vi "SDCP - Standard Message Frames Editor - Main.vi"() -> ()   [LabVIEW 2020]
uses:
  Typedefs/SDCP - Standard Message Frames Editor - Parameter cluster.ctl
panel:
  in  "Transmit tick (us)":dbl
  in  "Transmit code file path":path
  in  "Generator transmit code":bool
  in  "Load Excel File":bool
  in  "Source Excel file path":path
  in  "Destination Parameter file path":path
  in  "Parameter list":i32(listbox)
  in  "Parameter index":i32
  in  "Stop application":bool
  in  "Source Parameter file path":path
  in  "C code file path":path
  in  "Load parameter file":bool
  in  "Generate Parameter File":bool
  in  "Generate C code":bool
  in  "Frame ID":i32
  in  "Frame Name":string
  in  "Delete Parameter":bool
  in  "Frame details":T2(array[cluster])
  in  "Delete frame":bool
  in  "Add Frame":bool
  # "Frame Details"
  # "Note: \nValid data types for \nparameters are \nunsigned, signed and\nfloat."
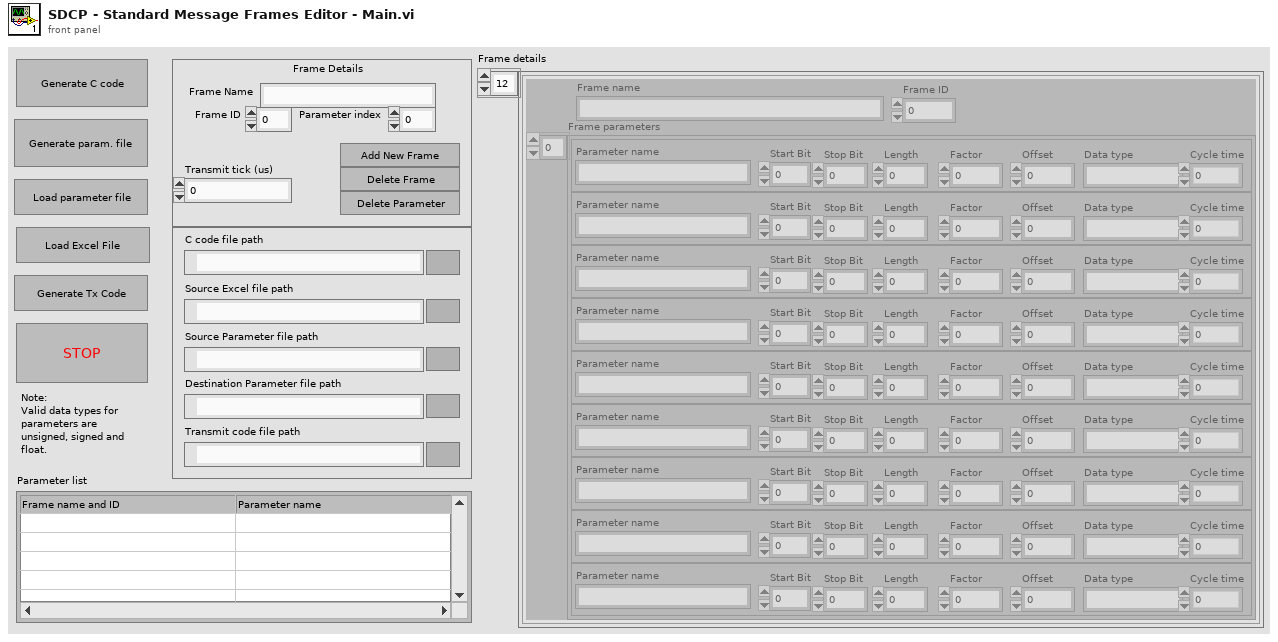
[diagram p1: front panel]
types:
  T1 = typedef "SDCP - Standard Message Frames Editor - Parameter cluster.ctl" = cluster{"Parameter name":string, "Start Bit":i32, "Stop Bit":i32, "Length":i32, "Factor":dbl, "Offset":dbl, "Data type":string, "Cycle time":dbl}
  T2 = cluster{"Frame name":string, "Frame ID":i32, "Frame parameters":T1[]}[]
  T3 = cluster{"Frame name":string, "Frame ID":i32, "Frame parameters":T1[]}
  T4 = enum16{"open", "replace", "create", "open or create", "replace or create", "replace or create with confirmation"}
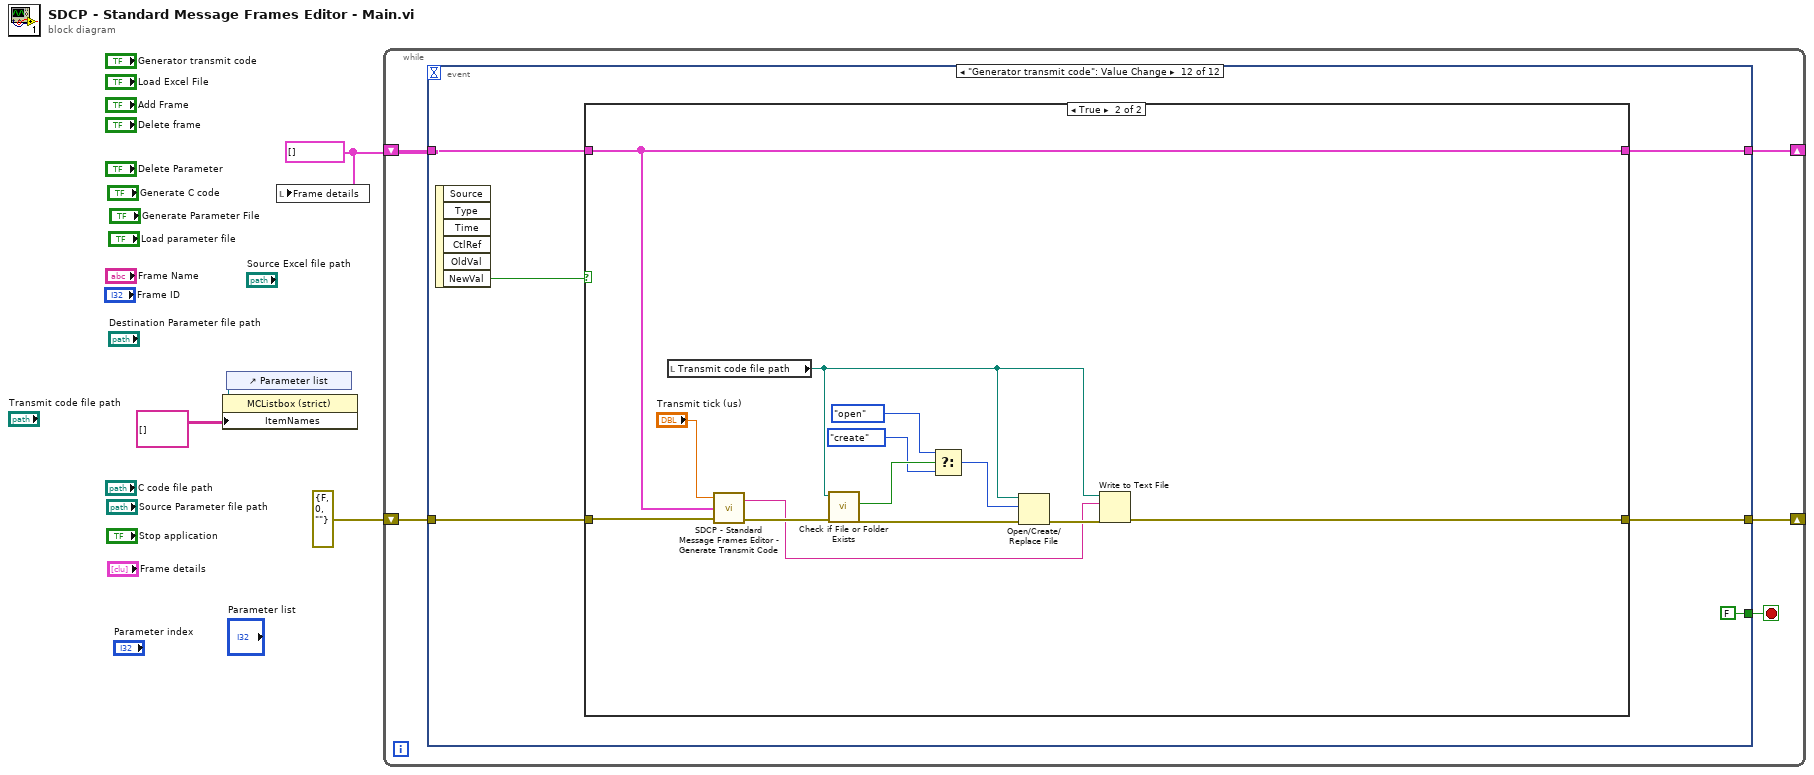
[diagram p0: block diagram]
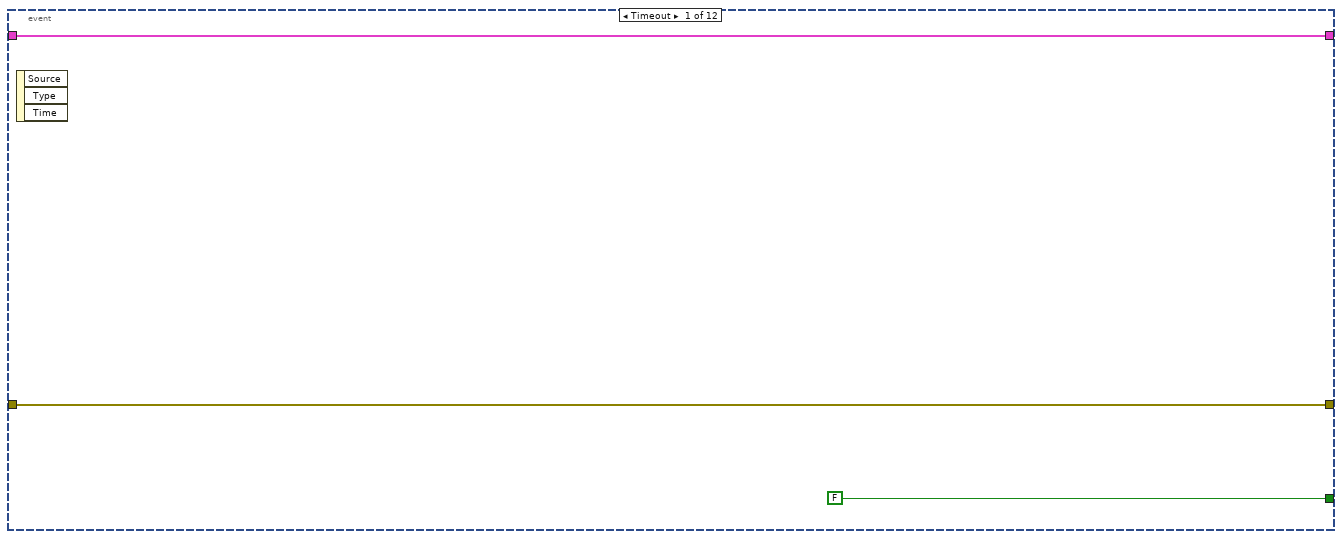
[diagram p2: hidden frame]
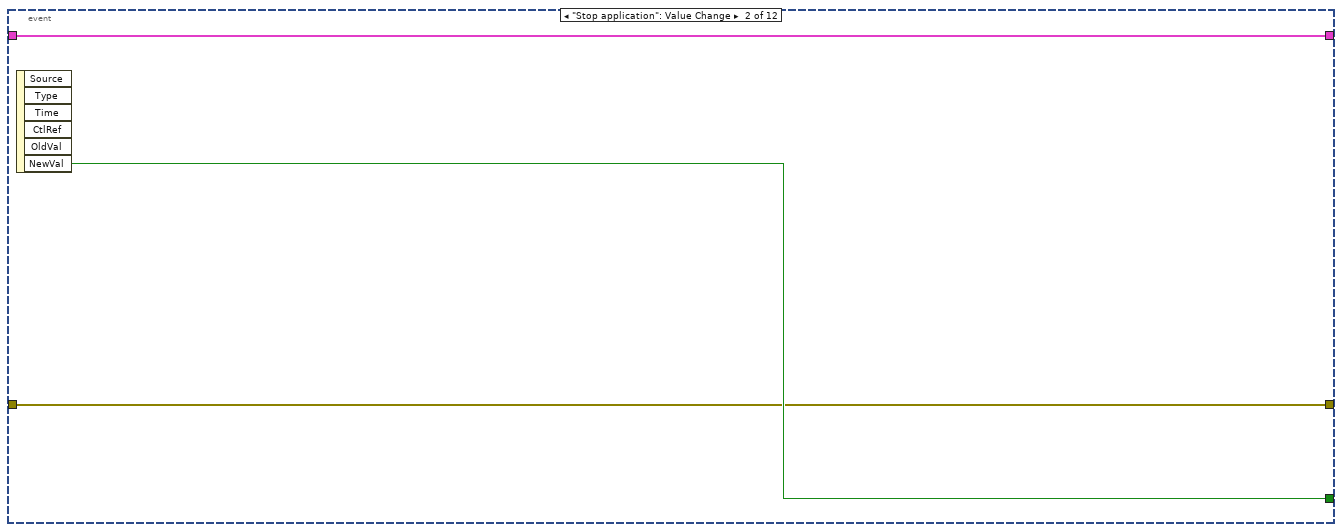
[diagram p3: hidden frame]
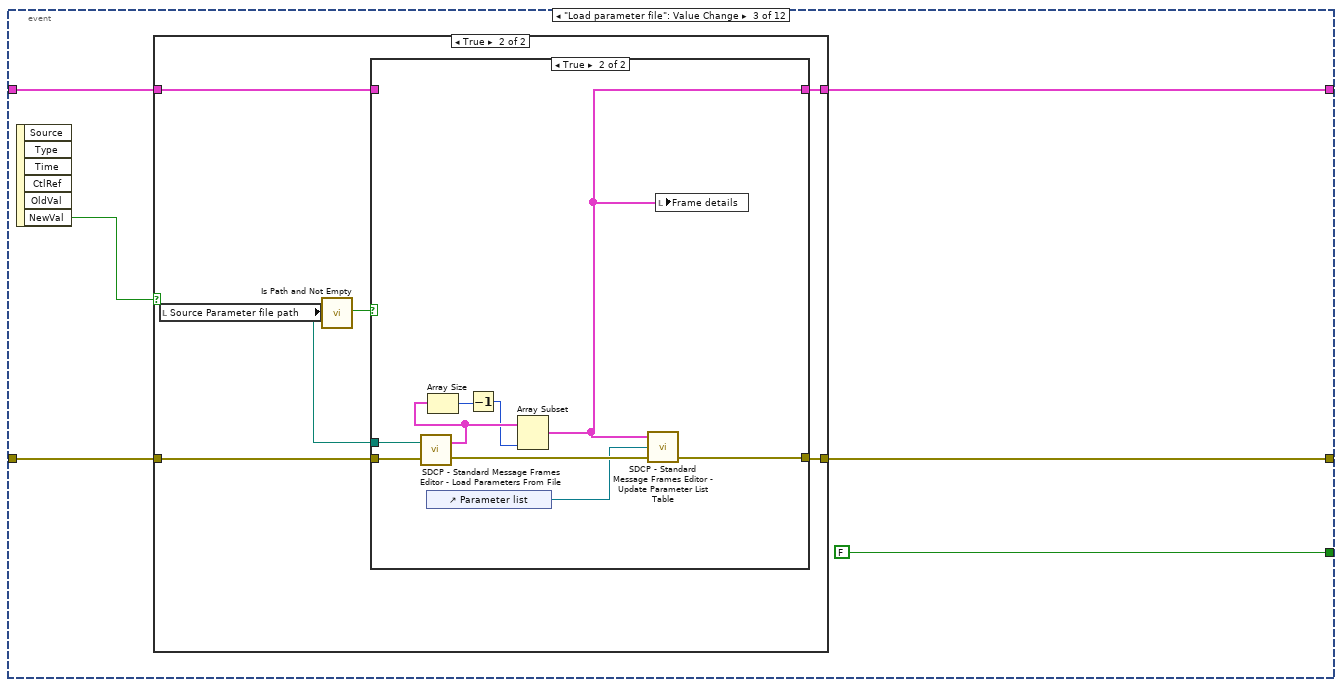
[diagram p4: hidden frame]
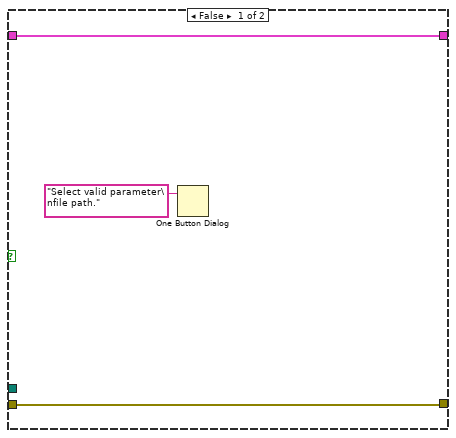
[diagram p6: hidden frame]
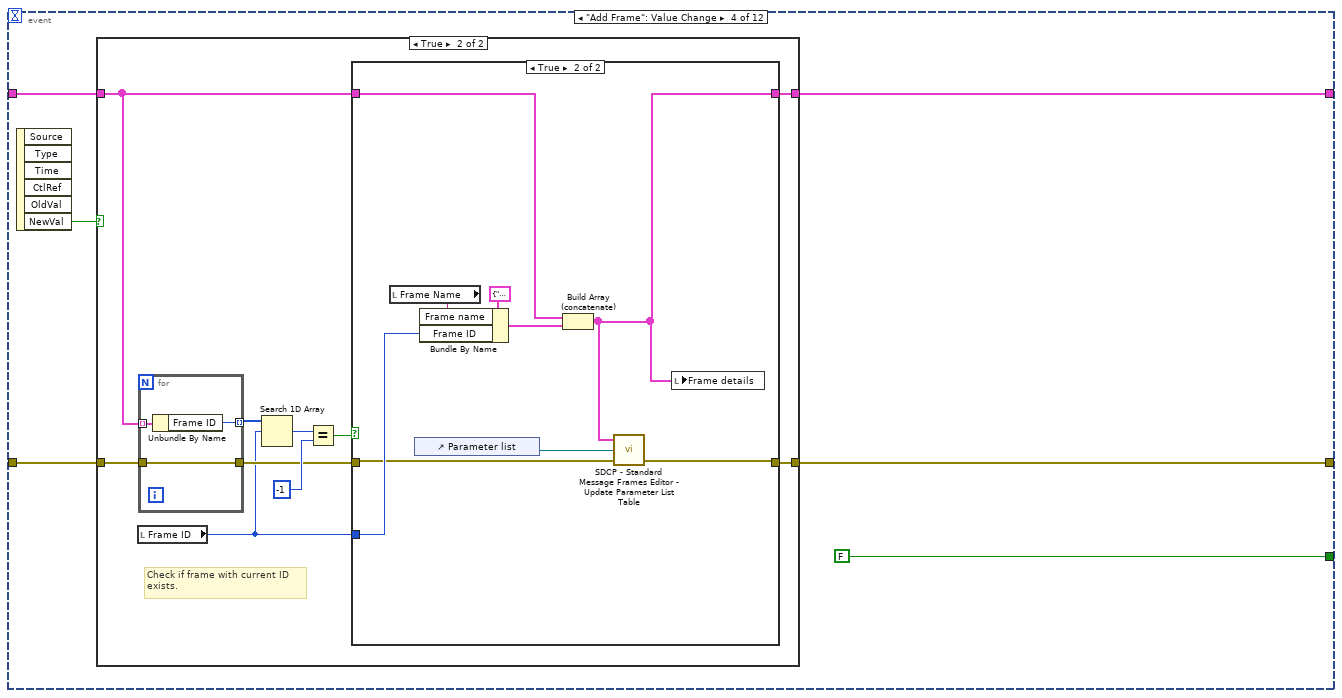
[diagram p7: hidden frame]
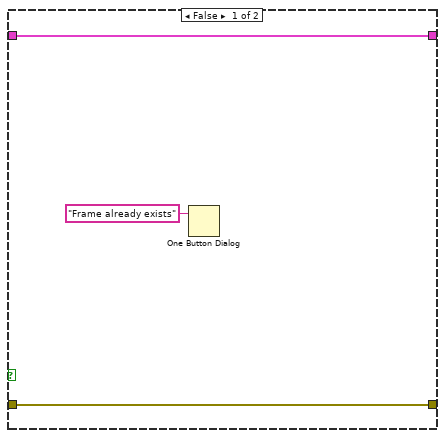
[diagram p9: hidden frame]
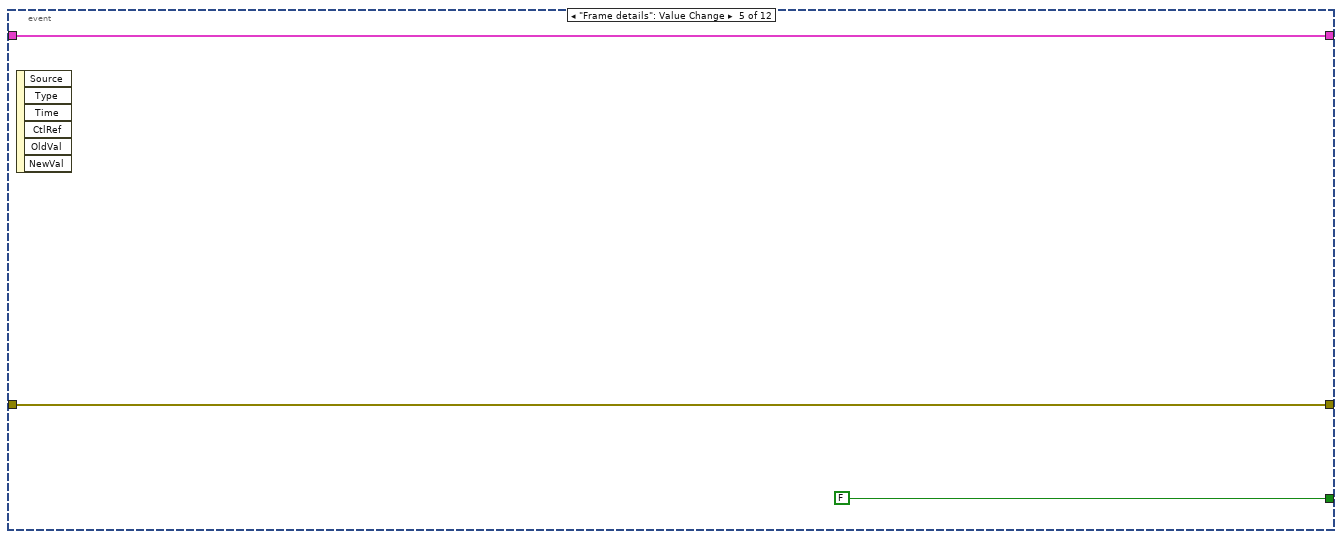
[diagram p10: hidden frame]
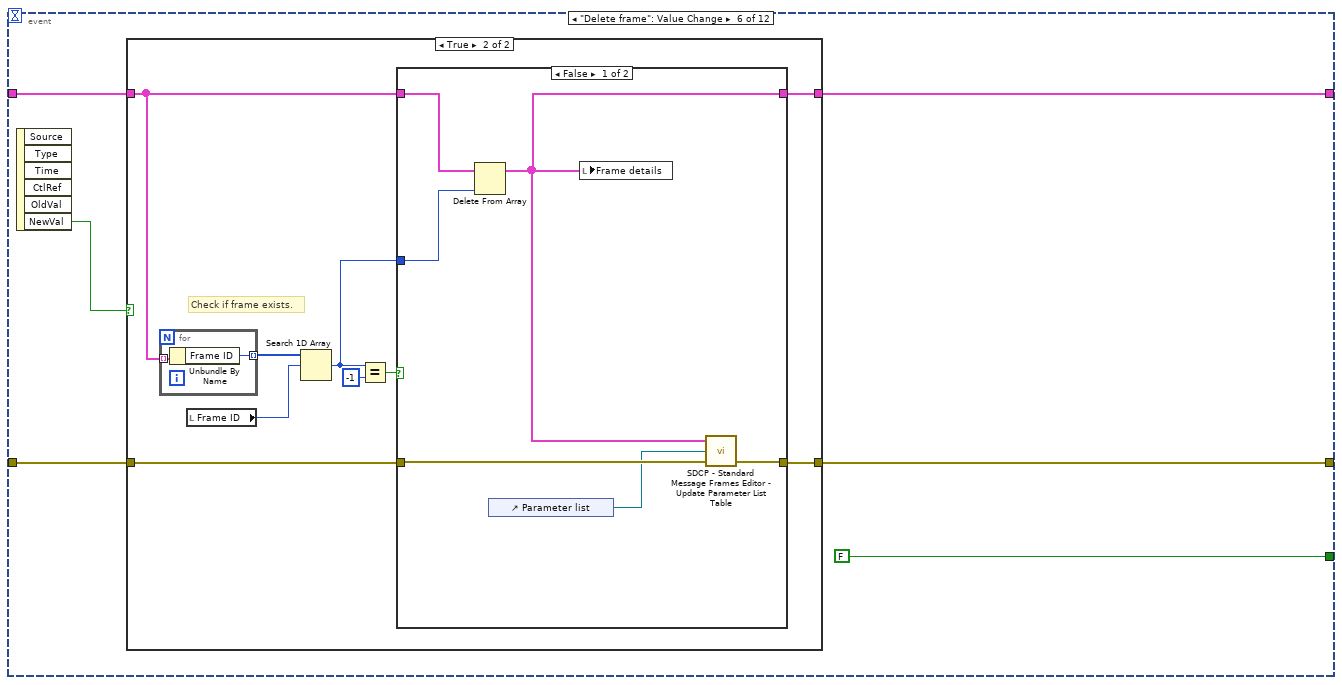
[diagram p11: hidden frame]
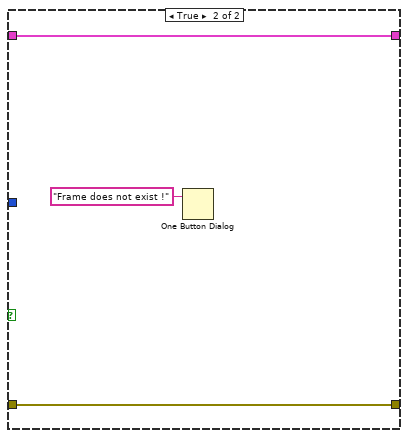
[diagram p13: hidden frame]
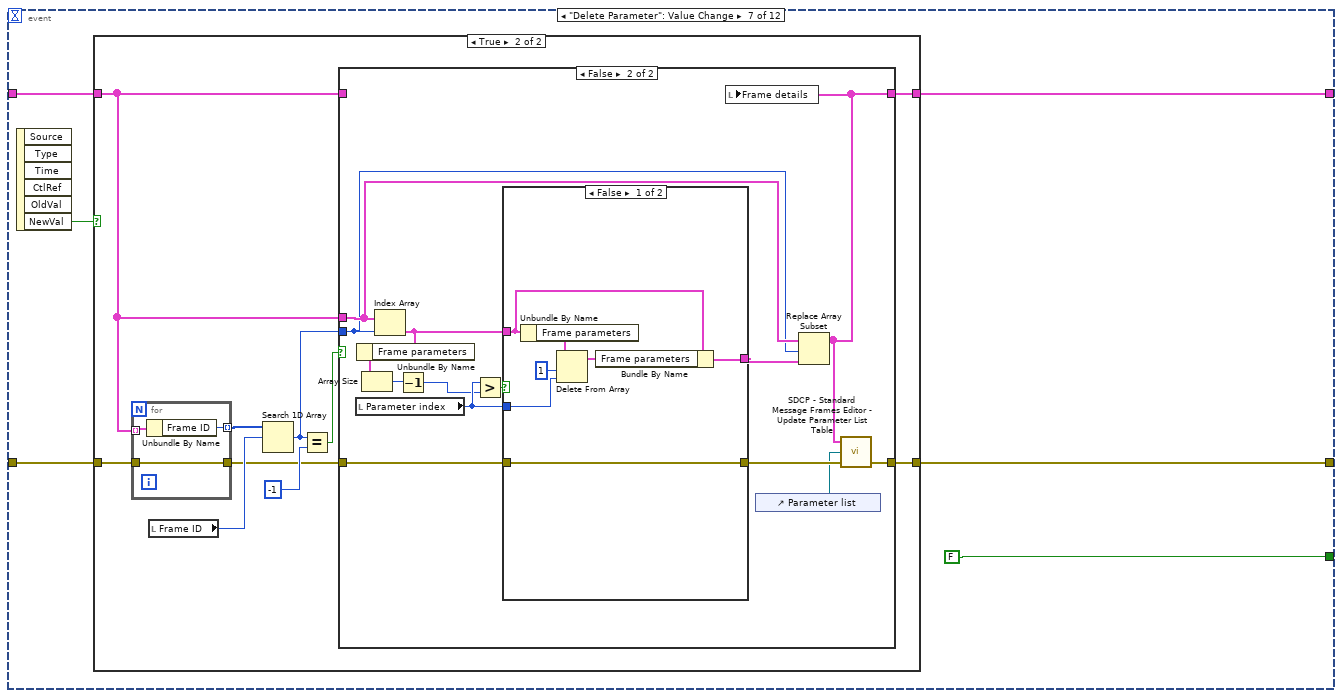
[diagram p14: hidden frame]
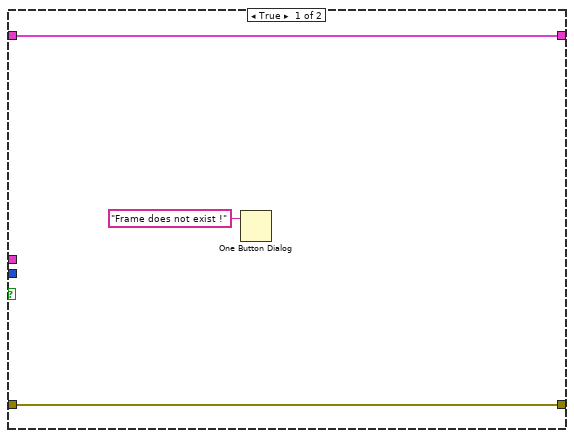
[diagram p16: hidden frame]
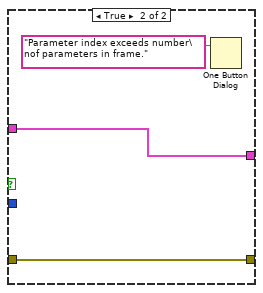
[diagram p17: hidden frame]
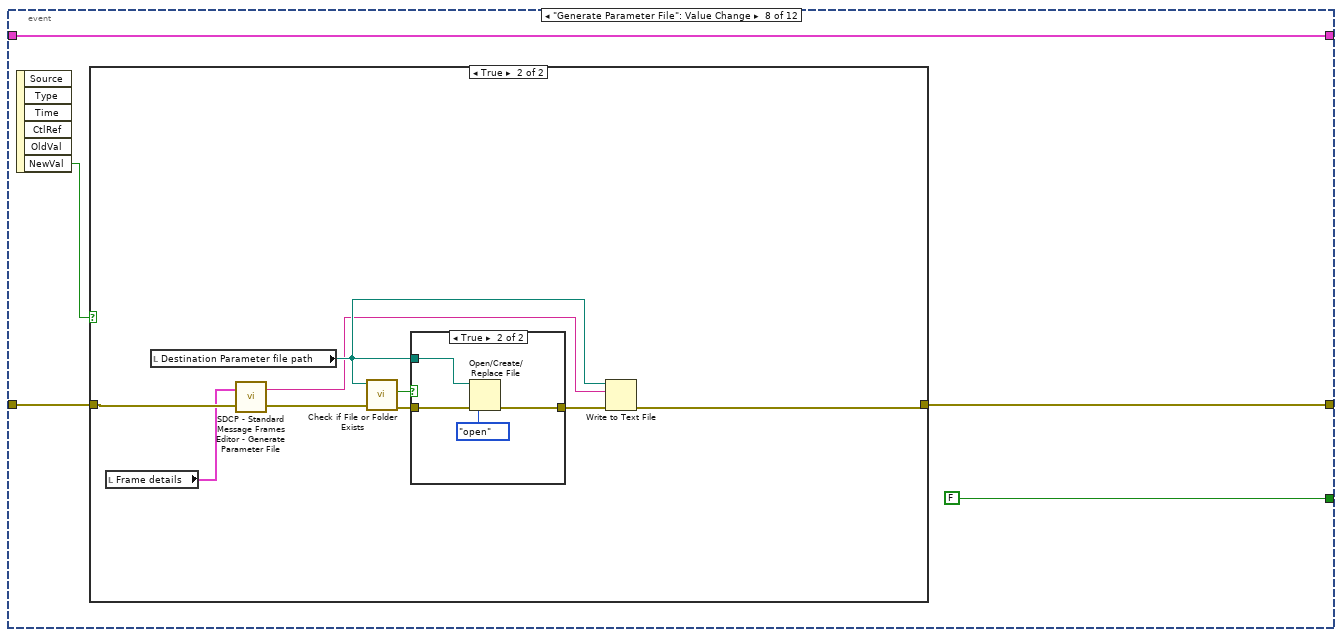
[diagram p18: hidden frame]
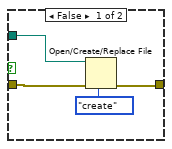
[diagram p20: hidden frame]
diagram:
  w3 = T2 []
  n1 = control-ref of="Parameter list"() -> (w2:refnum<vi>)
  n2 = property class="MCListbox (strict)"(reference=w2, "ItemNames"=string[][] []) -> ()  [unwired: 1 in, 2 out]
  n3 = local write "Frame details"(w3) -> ()
  n4 = while {
    shift-right: [w7] -> _
    shift-left: w3 -> [w8]
    shift-right: [w5] -> _
    shift-left: errorcluster {"status"=FALSE, "code"=0, "source"=""} ("error constant") -> [w6]
    stop <- w9 stop-if-true
    n5 = event shown="[11] \"Generator transmit code\": Value Change" {
      selector: _ -> [_ _ _ _ _ _ _ _ _ _ _ _]
      dyn-events: _ -> [_ _ _ _ _ _ _ _ _ _ _ _]
      timeout: _ -> [_ _ _ _ _ _ _ _ _ _ _ _]
      tunnel: [FALSE w15 FALSE ("NewVal") FALSE ("NewVal") FALSE ("NewVal") FALSE ("NewVal") FALSE ("NewVal") FALSE ("NewVal") FALSE ("NewVal") FALSE ("NewVal") FALSE ("NewVal") FALSE ("NewVal")] -> w9
      tunnel: w8 -> [w11 w14 w19 w43 w76 w79 w109 w154 w183 w216 w236 w248]
      tunnel: [w11 w14 w18 w42 w76 w78 w108 w154 w183 w216 w235 w247] -> w7
      tunnel: w6 -> [w10 w13 w20 w45 w75 w82 w107 w156 w201 w213 w239 w251]
      tunnel: [w10 w13 w16 w44 w75 w80 w106 w155 w200 w212 w237 w249] -> w5
      event Timeout {
        n6 = event-data() -> ()  [unwired: 1 in, 3 out]
      }
      event "Stop application": Value Change {
        n7 = event-data() -> ("NewVal"=w15:bool)  [unwired: 1 in, 5 out]
      }
      event "Load parameter file": Value Change {
        n8 = event-data() -> ("NewVal"=w17:bool)  [unwired: 1 in, 5 out]
        n9 = case shown="True" w17 {
          tunnel: w20 -> [w22 w29]
          tunnel: w19 -> [w23 w28]
          tunnel: [w23 w27] -> w18
          tunnel: [w22 w24] -> w16
          frame False {
          }
          frame True {
            n10 = local read "Source Parameter file path"() -> (w26:path)
            n11 = call <vilib>:"Is Path and Not Empty.vi"("path"=w26) -> ("Is Path and Not Empty?"=w25:bool)  [unwired: 4 in]
            n12 = case shown="True" w25 {
              tunnel: w29 -> [w31 w41]
              tunnel: w28 -> [w32 _]
              tunnel: [w32 w34] -> w27
              tunnel: [w31 w35] -> w24
              tunnel: w26 -> [_ w40]
              frame False {
                n13 = One Button Dialog(message="Select valid parameter\nfile path.") -> ()  [unwired: 1 in, 1 out]
              }
              frame True {
                n14 = call "SDCP - Standard Message Frames Editor - Load Parameters From File.vi"("error in (no error)"=w41, "Parameter File Path"=w40) -> ("error out"=w36:errorcluster, "Output"=w38:T2)
                n15 = control-ref of="Parameter list"() -> (w33:refnum<vi>)
                n16 = Array Size(array=w38) -> (size(s)=w39:i32)
                n17 = Decrement(x=w39) -> (x-1=w37:i32)
                n18 = Array Subset(array=w38, length=w37) -> (w34:T2)  [unwired: 1 in]
                n19 = call "SDCP - Standard Message Frames Editor - Update Parameter List Table.vi"("error in (no error)"=w36, "Listbox reference"=w33, "Input frame list"=w34) -> ("error out"=w35:errorcluster)  [unwired: 2 in]
                n20 = local write "Frame details"(w34) -> ()
              }
            }
          }
        }
      }
      event "Add Frame": Value Change {
        n21 = event-data() -> ("NewVal"=w46:bool)  [unwired: 1 in, 5 out]
        n22 = case shown="True" w46 {
          tunnel: w45 -> [w49 w59]
          tunnel: [w49 w51] -> w44
          tunnel: w43 -> [w48 w53]
          tunnel: [w48 w52] -> w42
          frame False {
          }
          frame True {
            # "Check if frame with current ID\nexists."
            n23 = local read "Frame ID"() -> (w50:i32)
            n24 = for {
              tunnel: w59 -> [w73]
              tunnel: w53 -> [w74] mode=indexing
              tunnel: [w73] -> w54
              tunnel: [w72] -> w58 mode=indexing
              n25 = Unbundle By Name(w74) -> ("Frame ID"=w72:i32)
            }
            n26 = Search 1D Array(1D array=w58, element=w50) -> (index of element=w57:i32)  [unwired: 1 in]
            n27 = Equal?(x=w57, y=-1) -> (x = y?=w55:bool)
            n28 = case shown="True" w55 {
              tunnel: w54 -> [w61 w66]
              tunnel: w53 -> [w62 w67]
              tunnel: [w62 w65] -> w52
              tunnel: [w61 w64] -> w51
              tunnel: w50 -> [_ w69]
              frame False {
                n29 = One Button Dialog(message="Frame already exists") -> ()  [unwired: 1 in, 1 out]
              }
              frame True {
                n30 = local read "Frame Name"() -> (w71:string)
                n31 = control-ref of="Parameter list"() -> (w63:refnum<vi>)
                n32 = Bundle By Name(cluster=T3 {"Frame name"="", "Frame ID"=0, "Frame parameters"=[]}, "Frame name"=w71, "Frame ID"=w69) -> (w68:T3)
                n33 = Build Array (concatenate)(w67, w68) -> (w65:T2)
                n34 = call "SDCP - Standard Message Frames Editor - Update Parameter List Table.vi"("error in (no error)"=w66, "Listbox reference"=w63, "Input frame list"=w65) -> ("error out"=w64:errorcluster)  [unwired: 2 in]
                n35 = local write "Frame details"(w65) -> ()
              }
            }
          }
        }
      }
      event "Frame details": Value Change {
        n36 = event-data() -> ()  [unwired: 1 in, 6 out]
      }
      event "Delete frame": Value Change {
        n37 = event-data() -> ("NewVal"=w81:bool)  [unwired: 1 in, 5 out]
        n38 = case shown="True" w81 {
          tunnel: w82 -> [w84 w91]
          tunnel: [w84 w90] -> w80
          tunnel: w79 -> [w85 w88]
          tunnel: [w85 w87] -> w78
          frame False {
          }
          frame True {
            # "Check if frame exists."
            n39 = for {
              tunnel: w88 -> [w105] mode=indexing
              tunnel: [w104] -> w94 mode=indexing
              n40 = Unbundle By Name(w105) -> ("Frame ID"=w104:i32)
            }
            n41 = local read "Frame ID"() -> (w93:i32)
            n42 = Search 1D Array(1D array=w94, element=w93) -> (index of element=w86:i32)  [unwired: 1 in]
            n43 = Equal?(x=w86, y=-1) -> (x = y?=w89:bool)
            n44 = case shown="False" w89 {
              tunnel: w91 -> [w98 w103]
              tunnel: [w97 w103] -> w90
              tunnel: w88 -> [w100 w102]
              tunnel: [w96 w102] -> w87
              tunnel: w86 -> [w99 _]
              frame False {
                n45 = Delete From Array(array=w100, index=w99) -> (array with subset deleted=w96:T2)  [unwired: 1 in, 1 out]
                n46 = control-ref of="Parameter list"() -> (w95:refnum<vi>)
                n47 = local write "Frame details"(w96) -> ()
                n48 = call "SDCP - Standard Message Frames Editor - Update Parameter List Table.vi"("error in (no error)"=w98, "Listbox reference"=w95, "Input frame list"=w96) -> ("error out"=w97:errorcluster)  [unwired: 2 in]
              }
              frame True {
                n49 = One Button Dialog(message="Frame does not exist !") -> ()  [unwired: 1 in, 1 out]
              }
            }
          }
        }
      }
      event "Delete Parameter": Value Change {
        n50 = event-data() -> ("NewVal"=w110:bool)  [unwired: 1 in, 5 out]
        n51 = case shown="True" w110 {
          tunnel: w109 -> [w113 w117]
          tunnel: [w113 w116] -> w108
          tunnel: w107 -> [w112 w123]
          tunnel: [w112 w115] -> w106
          frame False {
          }
          frame True {
            n52 = for {
              tunnel: w123 -> [w152]
              tunnel: w117 -> [w153] mode=indexing
              tunnel: [w152] -> w118
              tunnel: [w151] -> w122 mode=indexing
              n53 = Unbundle By Name(w153) -> ("Frame ID"=w151:i32)
            }
            n54 = local read "Frame ID"() -> (w121:i32)
            n55 = Search 1D Array(1D array=w122, element=w121) -> (index of element=w114:i32)  [unwired: 1 in]
            n56 = Equal?(x=w114, y=-1) -> (x = y?=w119:bool)
            n57 = case shown="False" w119 {
              tunnel: w118 -> [w125 w138]
              tunnel: w117 -> [_ w134]
              tunnel: w117 -> [w126 _]
              tunnel: [w126 w128] -> w116
              tunnel: [w125 w129] -> w115
              tunnel: w114 -> [_ w133]
              frame True {
                n58 = One Button Dialog(message="Frame does not exist !") -> ()  [unwired: 1 in, 1 out]
              }
              frame False {
                n59 = local read "Parameter index"() -> (w132:i32)
                n60 = Index Array(array=w134, index=w133) -> (element=w136:T3)
                n61 = Unbundle By Name(w136) -> ("Frame parameters"=w140:T1[])
                n62 = Array Size(array=w140) -> (size(s)=w139:i32)
                n63 = Decrement(x=w139) -> (x-1=w131:i32)
                n64 = Greater?(x=w132, y=w131) -> (0:w137:bool)
                n65 = case shown="False" w137 {
                  tunnel: w138 -> [w142 w150]
                  tunnel: [w142 w150] -> w130
                  tunnel: w136 -> [w144 w148]
                  tunnel: w132 -> [w145 _]
                  tunnel: [w141 w148] -> w135
                  frame False {
                    n66 = Unbundle By Name(w144) -> ("Frame parameters"=w147:T1[])
                    n67 = Delete From Array(array=w147, length=1, index=w145) -> (array with subset deleted=w143:T1[])  [unwired: 1 out]
                    n68 = Bundle By Name(cluster=w144, "Frame parameters"=w143) -> (w141:T3)
                  }
                  frame True {
                    n69 = One Button Dialog(message="Parameter index exceeds number\nof parameters in frame.") -> ()  [unwired: 1 in, 1 out]
                  }
                }
                n70 = control-ref of="Parameter list"() -> (w127:refnum<vi>)
                n71 = Replace Array Subset(array=w134, new element=w135, index=w133) -> (w128:T2)
                n72 = local write "Frame details"(w128) -> ()
                n73 = call "SDCP - Standard Message Frames Editor - Update Parameter List Table.vi"("error in (no error)"=w130, "Listbox reference"=w127, "Input frame list"=w128) -> ("error out"=w129:errorcluster)  [unwired: 2 in]
              }
            }
          }
        }
      }
      event "Generate Parameter File": Value Change {
        n74 = event-data() -> ("NewVal"=w157:bool)  [unwired: 1 in, 5 out]
        n75 = case shown="True" w157 {
          tunnel: w156 -> [w159 w168]
          tunnel: [w159 w161] -> w155
          frame False {
          }
          frame True {
            n76 = local read "Frame details"() -> (w160:T2)
            n77 = local read "Destination Parameter file path"() -> (w163:path)
            n78 = call "SDCP - Standard Message Frames Editor - Generate Parameter File.vi"("error in (no error)"=w168, "Frame details"=w160) -> ("error out"=w167:errorcluster, "Output"=w162:string)
            n79 = call <vilib>:"Check if File or Folder Exists.vi"("error in (no error)"=w167, "path"=w163) -> ("error out"=w165:errorcluster, "file or folder exists?"=w166:bool)  [unwired: 7 in, 1 out]
            n80 = case shown="True" w166 {
              tunnel: w165 -> [w172 w176]
              tunnel: [w169 w174] -> w164
              tunnel: w163 -> [w170 w175]
              frame False {
                n81 = Open/Create/Replace File(file path (use dialog)=w170, error in=w172, operation (0:open)=T4."create") -> (error out=w169:errorcluster)  [unwired: 3 in, 2 out]
              }
              frame True {
                n82 = Open/Create/Replace File(file path (use dialog)=w175, error in=w176, operation (0:open)=T4."open") -> (error out=w174:errorcluster)  [unwired: 3 in, 2 out]
              }
            }
            n83 = Write to Text File(file (use dialog)=w163, text=w162, error in=w164) -> (error out=w161:errorcluster)  [unwired: 1 in, 2 out]
          }
        }
      }
      event "Parameter list": Double Click {
        n84 = event-data() -> ("CtlRef"=w202:refnum<vi>, "Row"=w186:i32)  [unwired: 1 in, 7 out]
        n85 = property class="MCListbox (strict)"(reference=w202, error in=w201) -> (error out=w200:errorcluster, "ItemNames"=w188:string[][])  [unwired: 1 out]
        n86 = Increment(x=w186) -> (x+1=w195:i32)
        n87 = Index Array(array=w188, index (col)=0 ("disabled index (col)")) -> (element=w198:string[])  [unwired: 1 in]
        n88 = Index Array(array=w188, index (row)=w186, index (col)=1 ("disabled index (col)")) -> (element=w178:string)
        n89 = Array Subset(array=w198, length=w195) -> (w197:string[])  [unwired: 1 in]
        n90 = for {
          tunnel: w183 -> [w207] mode=indexing
          tunnel: [w206] -> w184 mode=indexing
          n91 = Unbundle By Name(w207) -> ("Frame ID"=w206:i32)
        }
        n92 = Reverse 1D Array(array=w197) -> (reversed array=w196:string[])
        n93 = while {
          tunnel: w196 -> [w209] mode=indexing
          tunnel: [w209] -> w193
          stop <- w210 stop-if-true
          n94 = call <vilib>:"Trim Whitespace.vi"("string"=w209) -> ("trimmed string"=w208:string)  [unwired: 1 in]
          n95 = Not Equal?(x="", y=w208) -> (x != y?=w210:bool)
        }
        n96 = Match Pattern(string=w193, regular expression="(") -> (before substring=w192:string, after substring=w191:string)  [unwired: 1 in, 2 out]
        n97 = Match Pattern(string=w191, regular expression=")") -> (before substring=w189:string)  [unwired: 1 in, 3 out]
        n98 = local write "Frame Name"(w192) -> ()
        n99 = Decimal String To Number(string=w189) -> (number=w185:i32)  [unwired: 2 in, 1 out]
        n100 = local write "Frame ID"(w185) -> ()
        n101 = Search 1D Array(1D array=w184, element=w185) -> (index of element=w182:i32)  [unwired: 1 in]
        n102 = Index Array(array=w183, index=w182) -> (element=w181:T3)
        n103 = Unbundle By Name(w181) -> ("Frame parameters"=w180:T1[])
        n104 = for {
          tunnel: w180 -> [w205] mode=indexing
          tunnel: [w204] -> w179 mode=indexing
          n105 = Unbundle By Name(w205) -> ("Parameter name"=w204:string)
        }
        n106 = Search 1D Array(1D array=w179, element=w178) -> (index of element=w177:i32)  [unwired: 1 in]
        n107 = local write "Parameter index"(w177) -> ()
      }
      event "Generate C code": Value Change {
        n108 = event-data() -> ("NewVal"=w214:bool)  [unwired: 1 in, 5 out]
        n109 = case shown="False" w214 {
          tunnel: w213 -> [w217 w226]
          tunnel: [w217 w218] -> w212
          frame False {
          }
          frame True {
            n110 = local read "Frame details"() -> (w225:T2)
            n111 = local read "C code file path"() -> (w220:path)
            n112 = call "SDCP - Standard Message Frames Editor - Generate C code.vi"("error in (no error)"=w226, "Frame details"=w225) -> ("error out"=w224:errorcluster, "Output"=w219:string)
            n113 = call <vilib>:"Check if File or Folder Exists.vi"("error in (no error)"=w224, "path"=w220) -> ("error out"=w222:errorcluster, "file or folder exists?"=w223:bool)  [unwired: 7 in, 1 out]
            n114 = case shown="True" w223 {
              tunnel: w222 -> [w230 w234]
              tunnel: w220 -> [w228 w233]
              tunnel: [w229 w231] -> w221
              frame False {
                n115 = Open/Create/Replace File(file path (use dialog)=w228, error in=w230, operation (0:open)=T4."create") -> (error out=w229:errorcluster)  [unwired: 3 in, 2 out]
              }
              frame True {
                n116 = Open/Create/Replace File(file path (use dialog)=w233, error in=w234, operation (0:open)=T4."open") -> (error out=w231:errorcluster)  [unwired: 3 in, 2 out]
              }
            }
            n117 = Write to Text File(file (use dialog)=w220, text=w219, error in=w221) -> (error out=w218:errorcluster)  [unwired: 1 in, 2 out]
          }
        }
      }
      event "Load Excel File": Value Change {
        n118 = event-data() -> ("NewVal"=w238:bool)  [unwired: 1 in, 5 out]
        n119 = case shown="True" w238 {
          tunnel: w239 -> [w242 w246]
          tunnel: [w242 w244] -> w237
          tunnel: w236 -> [w241 _]
          tunnel: [w241 w243] -> w235
          frame False {
          }
          frame True {
            n120 = local read "Source Excel file path"() -> (w245:path)
            n121 = call "SDCP - Standard Message Frames Editor - Load Excel File.vi"("error in (no error)"=w246, "Excel File Path"=w245) -> ("error out"=w244:errorcluster, "Parameters"=w243:T2)
            n122 = local write "Frame details"(w243) -> ()
          }
        }
      }
      event "Generator transmit code": Value Change {
        n123 = event-data() -> ("NewVal"=w250:bool)  [unwired: 1 in, 5 out]
        n124 = case shown="True" w250 {
          tunnel: w251 -> [w254 w267]
          tunnel: [w254 w257] -> w249
          tunnel: w248 -> [w253 w266]
          tunnel: [w253 w266] -> w247
          frame False {
          }
          frame True {
            n125 = local read "Transmit code file path"() -> (w256:path)
            n126 = call "SDCP - Standard Message Frames Editor - Generate Transmit Code.vi"("error in (no error)"=w267, "Frame details"=w266, "Transmit tick (us)"="Transmit tick (us)") -> ("error out"=w264:errorcluster, "Output"=w255:string)
            n127 = call <vilib>:"Check if File or Folder Exists.vi"("error in (no error)"=w264, "path"=w256) -> ("error out"=w262:errorcluster, "file or folder exists?"=w263:bool)  [unwired: 7 in, 1 out]
            n128 = Select(t=T4."open" ("operation (0:open)"), s=w263, f=T4."create" ("operation (0:open)")) -> (s? t:f=w259:T4)
            n129 = Open/Create/Replace File(file path (use dialog)=w256, error in=w262, operation (0:open)=w259) -> (error out=w258:errorcluster)  [unwired: 3 in, 2 out]
            n130 = Write to Text File(file (use dialog)=w256, text=w255, error in=w258) -> (error out=w257:errorcluster)  [unwired: 1 in, 2 out]
          }
        }
      }
    }
  }
